vi "SeqMgr.Generate Random ID.vi"() -> (0 "ID":string)   [LabVIEW 2024, in "EQMF.lvlib" / "SeqMgr.lvlib"]
uses:
  SeqMgr.lvlib
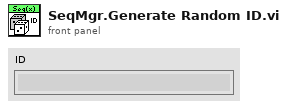
[diagram p1: front panel]
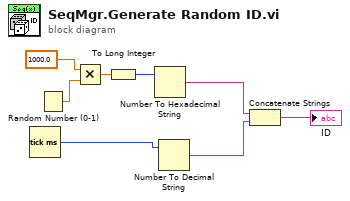
[diagram p0: block diagram]
diagram:
  n1 = Tick Count (ms)() -> (millisecond timer value=w3:u32)
  n2 = Random Number (0-1)() -> (number: 0 to 1=w5:dbl)
  n3 = Multiply(x=1000.0, y=w5) -> (x*y=w6:dbl)
  n4 = To Long Integer(number=w6) -> (32bit integer=w8:i32)
  n5 = Number To Hexadecimal String(2:w8) -> (0:w2:string)  [unwired: 1 in]
  n6 = Number To Decimal String(number=w3) -> (decimal integer string=w1:string)  [unwired: 1 in]
  n7 = Concatenate Strings(w2, w1) -> (→"ID":string)
